vi "SPC_set_parameter.vi"(6 "SPC parameter ID":T1 items=["CFD Limit Low", "CFD Limit High", "CFD Zero Cross Level", "CFD Holdoff", "SYNC Zero Cross Level", "SYNC Freq Divider", "SYNC Holdoff", "SYNC Threshold", "TAC Range", "TAC Gain", "TAC Offset", "TAC Limit Low", "TAC Limit High", "ADC Resolution", "External Latch Delay", "Collect Time", "Display Time", "Repeat Time", "Stop On Time", "Stop On Overflow", "Dither Range", "Count Increment", "Memory Bank", "Dead Time Compensation", "Scan Control", "Routing Mode", "TAC Enable Hold", "Operation Mode", "Scan Size X", "Scan Size Y", "Scan Routing X Bits", "Scan Routing Y Bits", "Scan Polarity", "Scan Flyback", "Scan Borders", "Pixel Time", "Pixel Clock Source", "Scan Line Compression", "External Trigger Condition", "External Pixel Clock Divider", "Rate Counting Time", "Macro Time Clock", "ADD Signal Source", "ADC Zoom", "XY Gain", "Image Size X", "Image Size Y", "Image Routing X Bits", "Image Routing Y Bits", "Master Clock", "ADC Sample Delay", "Detector Type", "X Axis Type", "Channel Enable", "Channel Slope", "Channel Spec_no", "TDC_OFFSET1", "TDC_OFFSET2", "TDC_OFFSET3", "TDC_OFFSET4"], 7 "Parameter Value":sgl format="%.2f", 8 "Error In":errorcluster, 10 "Module no":i16=-1 min=-1 max=7 step=1, 11 "DLL Path":path) -> (0 "Error Out":errorcluster, 2 "Module no":i16, 3 "DLL Path":path, 5 "Current Parameter Value":sgl format="%.2f")   [LabVIEW 2019]
doc: "The procedure sets the specified hardware parameter. The value of the specified parameter is transferred to the internal DLL structures of the module ‘mod_no’ and to the SPC module ‘mod_no’. \nIf ‘mod_no’ = -1, parameter will be changed for all SPC modules which are actually in use.\nThe new parameter value is recalculated according to the parameter limits, hardware restrictions (e.g. DAC resolution) and SPC module type. Furthermore, cross dependencies between different parameters are taken into account to ensure the correct hardware operation. \nIt is recommended to read back the parameters after setting it to get their real values after recalculation. This VI is actually calling SPC_get_parameter after the call to SPC_set_parameter to provide the actaual value after recalculation. But only if mod_no is not equal to -1.\nThe par_id values are defined in spcm_def.h file as SPC_PARAMETERS_KEYWORDS.\nLV users may use the type def /Public/Controls/par_id.ctl\n\ninfo@becker-hickl.com"
uses:
  SPC_Controls/par_id.ctl
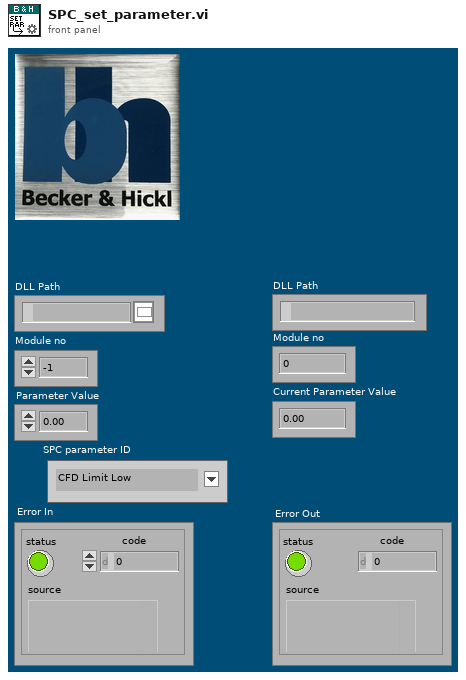
[diagram p1: front panel]
types:
  T1 = typedef "par_id.ctl" = i16
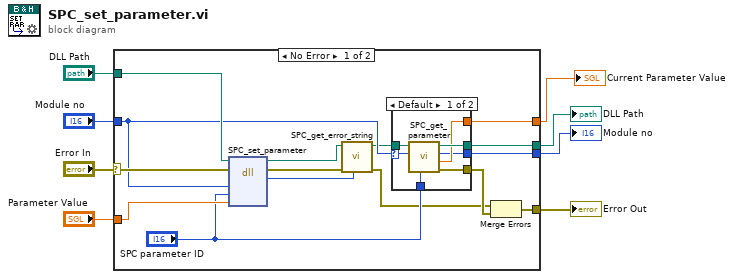
[diagram p0: block diagram]
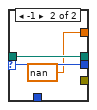
[diagram p2: hidden frame]
diagram:
  n1 = case shown="No Error" "Error In" {
    selector: "Error In" -> [w21 w37]
    tunnel: "DLL Path" -> [w23 w36]
    tunnel: [w22 w36] -> w7
    tunnel: [w10 w37] -> w6
    tunnel: "Module no" -> [w19 w35]
    tunnel: "Parameter Value" -> [w18 w34]
    tunnel: [w17 w34] -> w2
    tunnel: [w16 w35] -> w1
    frame No Error {
      n2 = dll-call lib="D:/spcm/lib/lab_view/lv10.0/spcm32.dll" fn="SPC_set_parameter"(path in=w23, error in=w21, "mod_no"=w19, "par_id"="SPC parameter ID", "value"=w18) -> (path out=w14:path, error out=w15:errorcluster, "return type"=w12:i16)  [unwired: 4 in]
      n3 = call "SPC_get_error_string.vi"("ErrorID"=w12, "Error In"=w15, "DLL Path"=w14) -> ("Error Out"=w9:errorcluster, "DLL Path"=w13:path)  [unwired: 6 in, 1 out]
      n4 = case shown="Default" w19 {
        selector: w19 -> [w28 w32]
        tunnel: [w30 w33] -> w22
        tunnel: [w29 _] -> w20
        tunnel: [w27 sgl nan ("Current Parameter Value")] -> w17
        tunnel: [w26 w32] -> w16
        tunnel: w13 -> [w25 w33]
        tunnel: "SPC parameter ID" -> [w24 _]
        frame Default {
          n5 = call "SPC_get_parameter.vi"("SPC Parameter ID"=w24, "Module No"=w28, "DLL Path"=w25) -> ("Error Out"=w29:errorcluster, "Current Parameter Value"=w27:sgl, "Module No"=w26:i16, "DLL Path"=w30:path)  [unwired: 5 in]
        }
        frame -1 {
        }
      }
      n6 = Merge Errors(w9, w20) -> (w10:errorcluster)
    }
    frame Error {
    }
  }
  "DLL Path" <- w7
  "Error Out" <- w6
  "Current Parameter Value" <- w2
  "Module no" <- w1
